vi "Evaluate Macro Command.vi"(8 "Error In":errorcluster, 10 "Cmd Index":i32, 11 "Macro Command String IN":string="LOOP.Start\t(loop.iterations,3.000);") -> (0 "Error Out":errorcluster, 1 "Warning?":bool, 2 "Macro Error Cluster":T1, 3 "Error in Command?":bool)   [LabVIEW 2012]
doc: "SciScan 1.2 160622"
uses:
  Macro Rule/subVIs/Error Checking/Macro Error Cluster.ctl
  INI/settingsIO/Settings IO_Commands.ctl
  FGV_MacroCore_Commands.ctl
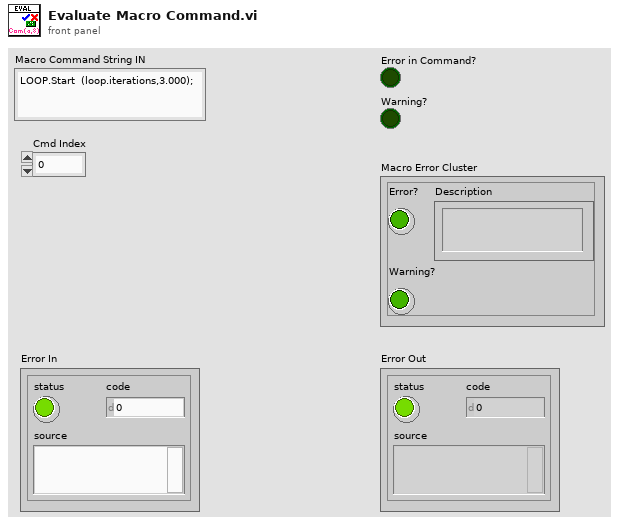
[diagram p1: front panel]
types:
  T1 = typedef "Macro Error Cluster.ctl" = cluster{"Error?":bool, "Description":string, "Warning?":bool}
  T2 = typedef "Settings IO_Commands.ctl" = enum16{"Write HW Settings", "Write Config Settings", "Read HW Settings", "Read Config Settings", "Write Line-Scan Settings", "Write Frame-Scan Settings", "Write Z-Stack Settings", "Read Line-Scan Settings", "Read Frame-Scan Settings", "Read Z-Stack Settings", "Read Fast-Z Settings", "Write Fast-Z Settings"}
  T3 = typedef "Macro_Action_List.ctl" = enum16{"Unknown Command", "2D.Frame.Scan", "2D.Line.Scan", "Load.Settings.File", "Move.To.Position", "Pause", "Z.Stack", "LOOP.Start", "LOOP.End", "Record", "Fast.Z", "Generic", "Slow.Z", "Tiling", "Preset.End"}
  T4 = typedef "GFG Variable for IO.ctl" = cluster{"Variable Name":string, "Value (Variant)":variant, "data type":string}
  T5 = typedef "FGV_MacroCore_Commands.ctl" = enum16{"Initialize", "Get Array", "Load macro from file", "Insert Item", "Insert at End", "Edit Parameter String", "Delete instruction", "Move Items", "Save", "SaveAs", "UpdateInfoTable", "Edit Settings File", "New Macro", "Read Temp File", "Delete Multiple"}
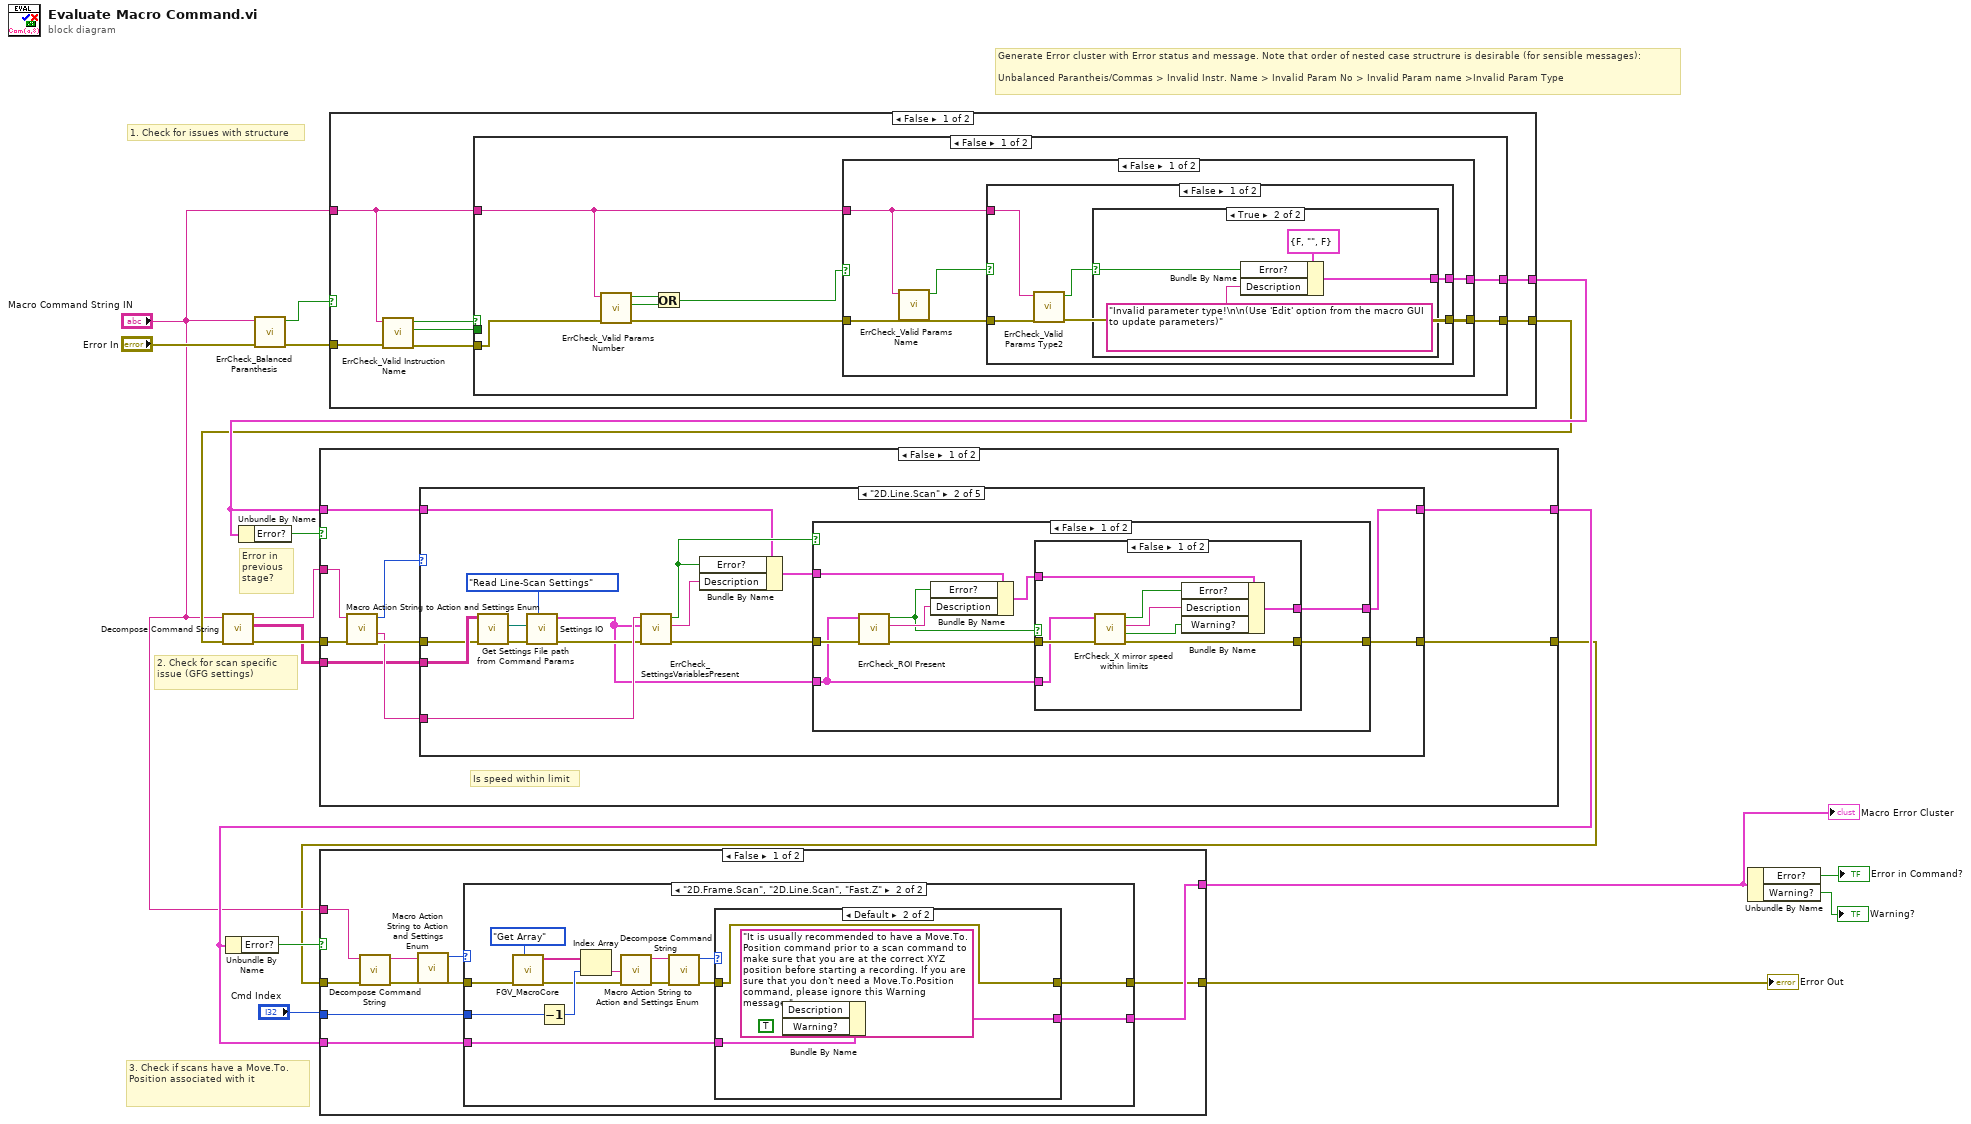
[diagram p0: block diagram]
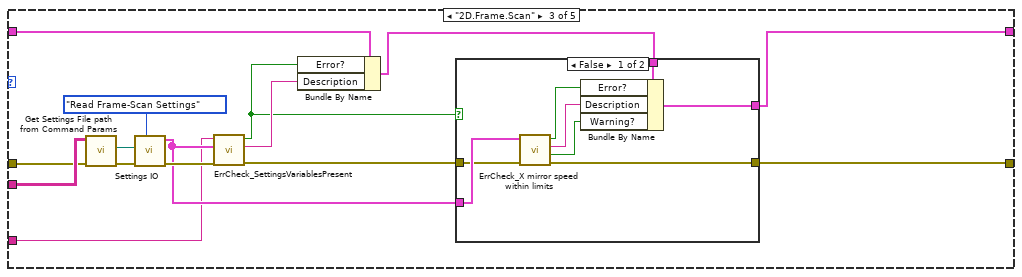
[diagram p8: hidden frame]
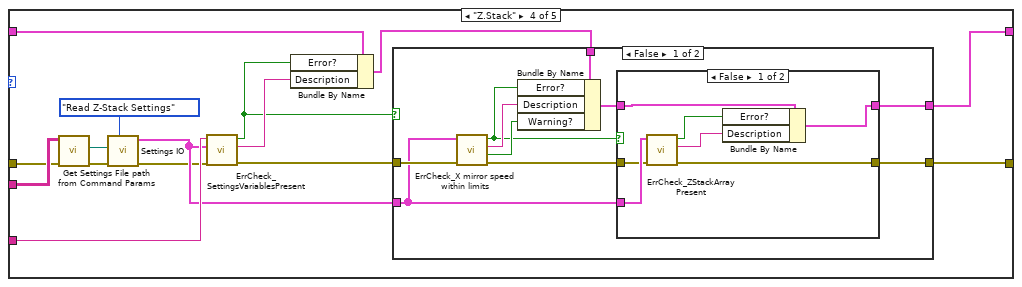
[diagram p10: hidden frame]
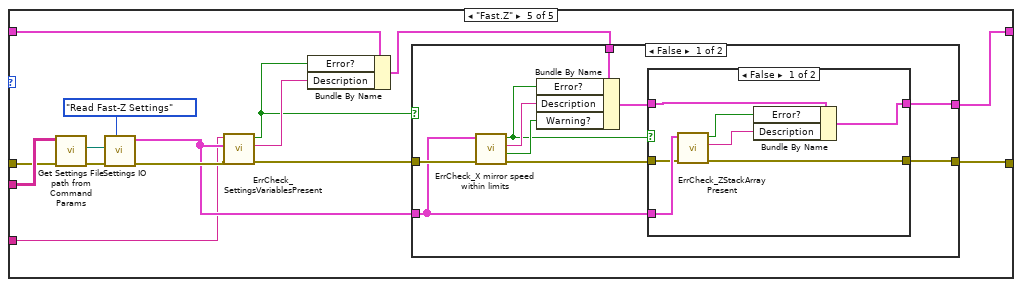
[diagram p13: hidden frame]
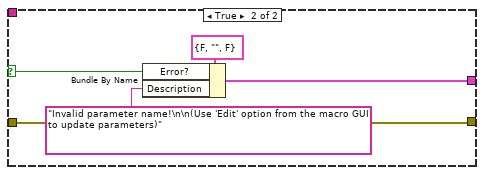
[diagram p18: hidden frame]
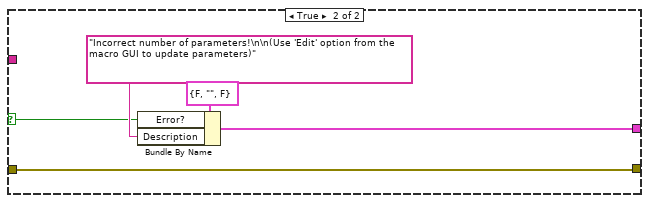
[diagram p19: hidden frame]
diagram:
  # "3. Check if scans have a Move.To.Position associated with it"
  # "2. Check for scan specific issue (GFG settings)"
  # "Error in previous stage?"
  # "1. Check for issues with structure"
  # "Generate Error cluster with Error status and message. Note that order of nested case structrure is desirable (for sensible messages):\n\nUnbalanced Parantheis/Commas > Invalid Instr. Name > Invalid Param No > Invalid Param name >Invalid Param Type"
  n1 = call "ErrCheck_Balanced Paranthesis.vi"("Error In"="Error In", "Macro Command String IN"="Macro Command String IN") -> ("Error Out"=w17:errorcluster, "Unbalanced Paranthesis or Commas?"=w16:bool)  [unwired: 8 in]
  n2 = case shown="False" w16 {
    selector: w16 -> [_ w68]
    tunnel: "Macro Command String IN" -> [w25 _]
    tunnel: [w24 w66] -> w11
    tunnel: w17 -> [w23 w66]
    tunnel: [w21 w67] -> w13
    frame False {
      n3 = call "ErrCheck_Valid Instruction Name.vi"("Error In"=w23, "Macro Command String IN"=w25) -> ("Error Out"=w22:errorcluster, "Generic Instruction?"=w20:bool, "Invalid Instruction name?"=w19:bool)  [unwired: 7 in]
      n4 = case shown="False" w19 {
        selector: w19 -> [_ w60]
        tunnel: w25 -> [w33 _]
        tunnel: [w31 w58] -> w24
        tunnel: w22 -> [w30 w58]
        tunnel: [w26 w61] -> w21
        tunnel: w20 -> [_ w59]
        frame False {
          n5 = call "ErrCheck_Valid Params Number.vi"("Error In"=w30, "Macro Command String IN"=w33) -> ("Error Out"=w27:errorcluster, "Less params than expected?"=w28:bool, "More params than expected?"=w29:bool)  [unwired: 7 in]
          n6 = Or(x=w29, y=w28) -> (x .or. y?=w32:bool)
          n7 = case shown="False" w32 {
            selector: w32 -> [_ w55]
            tunnel: w33 -> [w34 _]
            tunnel: [w38 w53] -> w31
            tunnel: w27 -> [w37 w53]
            tunnel: [w35 w54] -> w26
            frame False {
              n8 = call "ErrCheck_Valid Params Name.vi"("Macro Command String IN"=w34) -> ("Invalid Params name?"=w36:bool)  [unwired: 9 in, 1 out]
              n9 = case shown="False" w36 {
                selector: w36 -> [_ w50]
                tunnel: w34 -> [w43 _]
                tunnel: [w42 w48] -> w38
                tunnel: w37 -> [w41 w48]
                tunnel: [w39 w49] -> w35
                frame False {
                  n10 = call "ErrCheck_Valid Params Type2.vi"("Error In"=w41, "Macro Command String IN"=w43) -> ("Error Out"=w42:errorcluster, "Invalid params type?"=w40:bool)  [unwired: 8 in]
                  n11 = case shown="True" w40 {
                    selector: w40 -> [_ w45]
                    tunnel: [_ w44] -> w39
                    frame False {
                    }
                    frame True {
                      n12 = Bundle By Name(cluster=T1 {"Error?"=FALSE, "Description"="", "Warning?"=FALSE} ("Macro Error Cluster"), "Error?"=w45, "Description"="Invalid parameter type!\n\n(Use 'Edit' option from the macro GUI to update parameters)") -> (w44:T1)
                    }
                  }
                }
                frame True {
                  n13 = Bundle By Name(cluster=T1 {"Error?"=FALSE, "Description"="", "Warning?"=FALSE} ("Macro Error Cluster"), "Error?"=w50, "Description"="Invalid parameter name!\n\n(Use 'Edit' option from the macro GUI to update parameters)") -> (w49:T1)
                }
              }
            }
            frame True {
              n14 = Bundle By Name(cluster=T1 {"Error?"=FALSE, "Description"="", "Warning?"=FALSE} ("Macro Error Cluster"), "Error?"=w55, "Description"="Incorrect number of parameters!\n\n(Use 'Edit' option from the macro GUI to update parameters)") -> (w54:T1)
            }
          }
        }
        frame True {
          n15 = case shown="True" w59 {
            tunnel: [w65 _] -> w61
            tunnel: w60 -> [w62 _]
            frame False {
              n16 = Bundle By Name(cluster=T1 {"Error?"=FALSE, "Description"="", "Warning?"=FALSE} ("Macro Error Cluster"), "Error?"=w62, "Description"="Invalid instruction name!\n\nDelete the instruction (drag and drop it into available actions), and add the instruction you want again") -> (w65:T1)
            }
            frame True {
            }
          }
        }
      }
    }
    frame True {
      n17 = Bundle By Name(cluster=T1 {"Error?"=FALSE, "Description"="", "Warning?"=FALSE} ("Macro Error Cluster"), "Error?"=w68, "Description"="Unbalanced parantheis or 'parameter-value' pairs!\n\n(Use 'Edit' option from the macro GUI to update parameters)") -> (w67:T1)
    }
  }
  n18 = call "Decompose Command String.vi"("Error In"=w11, "Command IN"="Macro Command String IN") -> ("Error Out"=w10:errorcluster, "Parameter Table"=w9:string[][], "Action"=w12:string)  [unwired: 6 in, 1 out]
  n19 = Unbundle By Name(w13) -> ("Error?"=w14:bool)
  n20 = case shown="False" w14 {
    tunnel: w10 -> [w77 w215]
    tunnel: w12 -> [w76 _]
    tunnel: w13 -> [w78 w216]
    tunnel: [w79 w216] -> w6
    tunnel: w9 -> [w72 _]
    tunnel: [w71 w215] -> w3
    frame False {
      # "Is speed within limit"
      n21 = call "Macro Action String to Action and Settings Enum.vi"("error in (no error)"=w77, "Action String IN"=w76) -> ("error out"=w74:errorcluster, "Settings File Type OUT (String)"=w73:string, "Action Enum OUT"=w75:T3)  [unwired: 6 in, 1 out]
      n22 = case shown="\"2D.Line.Scan\"" w75 {
        tunnel: [w81 w83 w127 w145 w180] -> w79
        tunnel: w78 -> [w81 w86 w120 w146 w182]
        tunnel: w74 -> [w80 w92 w128 w153 w189]
        tunnel: w73 -> [_ w91 w122 w148 w181]
        tunnel: w72 -> [_ w95 w131 w156 w192]
        tunnel: [w80 w82 w126 w144 w179] -> w71
        frame "Unknown Command", Default {
        }
        frame "2D.Line.Scan" {
          n23 = call "Get Settings File path from Command Params.vi"("error in (no error)"=w92, "Params Array IN"=w95) -> ("error out"=w93:errorcluster, "Settings Path OUT"=w94:path)  [unwired: 8 in]
          n24 = call "Settings IO.vi"("SettingsFileIO_Commands"=Settings_IO_Commands."Read Line-Scan Settings", "Error In"=w93, "File Path (for scan specific settings)"=w94) -> ("Error Out"=w89:errorcluster, "Settings Array OUT"=w87:T4[])  [unwired: 6 in, 1 out]
          n25 = call "ErrCheck_SettingsVariablesPresent.vi"("error in (no error)"=w89, "Settings Array IN"=w87, "Settings type string"=w91) -> ("error out"=w84:errorcluster, "Error String"=w90:string, "Error?"=w88:bool)  [unwired: 6 in]
          n26 = Bundle By Name(cluster=w86, "Error?"=w88, "Description"=w90) -> (w85:T1)
          n27 = case shown="False" w88 {
            tunnel: w87 -> [w99 _]
            tunnel: w85 -> [w104 w117]
            tunnel: w84 -> [w101 w116]
            tunnel: [w98 w117] -> w83
            tunnel: [w97 w116] -> w82
            frame False {
              n28 = call "ErrCheck_ROI Present.vi"("Error In"=w101, "Settings ArrayIN"=w99) -> ("Error Out"=w100:errorcluster, "Error/Warning Message"=w105:string, "ROI Descriptor Missing?"=w103:bool)  [unwired: 7 in]
              n29 = Bundle By Name(cluster=w104, "Error?"=w103, "Description"=w105) -> (w102:T1)
              n30 = case shown="False" w103 {
                tunnel: w102 -> [w110 w115]
                tunnel: w100 -> [w109 w114]
                tunnel: w99 -> [w108 _]
                tunnel: [w107 w115] -> w98
                tunnel: [w106 w114] -> w97
                frame False {
                  n31 = call "ErrCheck_X mirror speed within limits.vi"("Error In"=w109, "Settings ArrayIN"=w108) -> ("Error Out"=w106:errorcluster, "Not Enough Variables (Warning)?"=w112:bool, "Error/Warning Message"=w113:string, "Speed  out of Limits?"=w111:bool)  [unwired: 6 in]
                  n32 = Bundle By Name(cluster=w110, "Error?"=w111, "Description"=w113, "Warning?"=w112) -> (w107:T1)
                }
                frame True {
                }
              }
            }
            frame True {
            }
          }
        }
        frame "2D.Frame.Scan" {
          n33 = call "Get Settings File path from Command Params.vi"("error in (no error)"=w128, "Params Array IN"=w131) -> ("error out"=w129:errorcluster, "Settings Path OUT"=w130:path)  [unwired: 8 in]
          n34 = call "Settings IO.vi"("SettingsFileIO_Commands"=Settings_IO_Commands."Read Frame-Scan Settings", "Error In"=w129, "File Path (for scan specific settings)"=w130) -> ("Error Out"=w124:errorcluster, "Settings Array OUT"=w123:T4[])  [unwired: 6 in, 1 out]
          n35 = call "ErrCheck_SettingsVariablesPresent.vi"("error in (no error)"=w124, "Settings Array IN"=w123, "Settings type string"=w122) -> ("error out"=w121:errorcluster, "Error String"=w125:string, "Error?"=w118:bool)  [unwired: 6 in]
          n36 = Bundle By Name(cluster=w120, "Error?"=w118, "Description"=w125) -> (w119:T1)
          n37 = case shown="False" w118 {
            tunnel: w121 -> [w136 w141]
            tunnel: w123 -> [w137 _]
            tunnel: w119 -> [w134 w142]
            tunnel: [w133 w142] -> w127
            tunnel: [w135 w141] -> w126
            frame False {
              n38 = call "ErrCheck_X mirror speed within limits.vi"("Error In"=w136, "Settings ArrayIN"=w137) -> ("Error Out"=w135:errorcluster, "Not Enough Variables (Warning)?"=w139:bool, "Error/Warning Message"=w138:string, "Speed  out of Limits?"=w140:bool)  [unwired: 6 in]
              n39 = Bundle By Name(cluster=w134, "Error?"=w140, "Description"=w138, "Warning?"=w139) -> (w133:T1)
            }
            frame True {
            }
          }
        }
        frame "Z.Stack" {
          n40 = call "Get Settings File path from Command Params.vi"("error in (no error)"=w153, "Params Array IN"=w156) -> ("error out"=w154:errorcluster, "Settings Path OUT"=w155:path)  [unwired: 8 in]
          n41 = call "Settings IO.vi"("SettingsFileIO_Commands"=Settings_IO_Commands."Read Z-Stack Settings", "Error In"=w154, "File Path (for scan specific settings)"=w155) -> ("Error Out"=w143:errorcluster, "Settings Array OUT"=w147:T4[])  [unwired: 6 in, 1 out]
          n42 = call "ErrCheck_SettingsVariablesPresent.vi"("error in (no error)"=w143, "Settings Array IN"=w147, "Settings type string"=w148) -> ("error out"=w151:errorcluster, "Error String"=w152:string, "Error?"=w149:bool)  [unwired: 6 in]
          n43 = Bundle By Name(cluster=w146, "Error?"=w149, "Description"=w152) -> (w150:T1)
          n44 = case shown="False" w149 {
            tunnel: w151 -> [w165 w177]
            tunnel: w147 -> [w160 _]
            tunnel: w150 -> [w164 w178]
            tunnel: [w161 w178] -> w145
            tunnel: [w158 w177] -> w144
            frame False {
              n45 = call "ErrCheck_X mirror speed within limits.vi"("Error In"=w165, "Settings ArrayIN"=w160) -> ("Error Out"=w159:errorcluster, "Not Enough Variables (Warning)?"=w167:bool, "Error/Warning Message"=w166:string, "Speed  out of Limits?"=w163:bool)  [unwired: 6 in]
              n46 = Bundle By Name(cluster=w164, "Error?"=w163, "Description"=w166, "Warning?"=w167) -> (w162:T1)
              n47 = case shown="False" w163 {
                tunnel: w162 -> [w172 w176]
                tunnel: [w168 w176] -> w161
                tunnel: w160 -> [w174 _]
                tunnel: w159 -> [w173 w175]
                tunnel: [w169 w175] -> w158
                frame False {
                  n48 = call "ErrCheck_ZStackArray Present.vi"("Error In"=w173, "Settings ArrayIN"=w174) -> ("Error Out"=w169:errorcluster, "Error/Warning Message"=w170:string, "Z-Stack data missing?"=w171:bool)  [unwired: 7 in]
                  n49 = Bundle By Name(cluster=w172, "Error?"=w171, "Description"=w170) -> (w168:T1)
                }
                frame True {
                }
              }
            }
            frame True {
            }
          }
        }
        frame "Fast.Z" {
          n50 = call "Get Settings File path from Command Params.vi"("error in (no error)"=w189, "Params Array IN"=w192) -> ("error out"=w190:errorcluster, "Settings Path OUT"=w191:path)  [unwired: 8 in]
          n51 = call "Settings IO.vi"("SettingsFileIO_Commands"=Settings_IO_Commands."Read Fast-Z Settings", "Error In"=w190, "File Path (for scan specific settings)"=w191) -> ("Error Out"=w184:errorcluster, "Settings Array OUT"=w183:T4[])  [unwired: 6 in, 1 out]
          n52 = call "ErrCheck_SettingsVariablesPresent.vi"("error in (no error)"=w184, "Settings Array IN"=w183, "Settings type string"=w181) -> ("error out"=w187:errorcluster, "Error String"=w188:string, "Error?"=w185:bool)  [unwired: 6 in]
          n53 = Bundle By Name(cluster=w182, "Error?"=w185, "Description"=w188) -> (w186:T1)
          n54 = case shown="False" w185 {
            tunnel: w187 -> [w201 w213]
            tunnel: w183 -> [w198 _]
            tunnel: w186 -> [w200 w214]
            tunnel: [w196 w214] -> w180
            tunnel: [w195 w213] -> w179
            frame False {
              n55 = call "ErrCheck_X mirror speed within limits.vi"("Error In"=w201, "Settings ArrayIN"=w198) -> ("Error Out"=w199:errorcluster, "Not Enough Variables (Warning)?"=w203:bool, "Error/Warning Message"=w202:string, "Speed  out of Limits?"=w194:bool)  [unwired: 6 in]
              n56 = Bundle By Name(cluster=w200, "Error?"=w194, "Description"=w202, "Warning?"=w203) -> (w197:T1)
              n57 = case shown="False" w194 {
                tunnel: w197 -> [w208 w212]
                tunnel: [w204 w212] -> w196
                tunnel: w198 -> [w210 _]
                tunnel: w199 -> [w209 w211]
                tunnel: [w205 w211] -> w195
                frame False {
                  n58 = call "ErrCheck_ZStackArray Present.vi"("Error In"=w209, "Settings ArrayIN"=w210) -> ("Error Out"=w205:errorcluster, "Error/Warning Message"=w206:string, "Z-Stack data missing?"=w207:bool)  [unwired: 7 in]
                  n59 = Bundle By Name(cluster=w208, "Error?"=w207, "Description"=w206) -> (w204:T1)
                }
                frame True {
                }
              }
            }
            frame True {
            }
          }
        }
      }
    }
    frame True {
    }
  }
  n60 = Unbundle By Name(w6) -> ("Error?"=w7:bool)
  n61 = case shown="False" w7 {
    tunnel: [w218 w251] -> w2
    tunnel: w6 -> [w219 w251]
    tunnel: "Cmd Index" -> [w226 _]
    tunnel: "Macro Command String IN" -> [w225 _]
    tunnel: w3 -> [w221 w250]
    tunnel: [w217 w250] -> w1
    frame False {
      n62 = call "Decompose Command String.vi"("Error In"=w221, "Command IN"=w225) -> ("Error Out"=w222:errorcluster, "Action"=w224:string)  [unwired: 6 in, 2 out]
      n63 = call "Macro Action String to Action and Settings Enum.vi"("error in (no error)"=w222, "Action String IN"=w224) -> ("error out"=w220:errorcluster, "Action Enum OUT"=w223:T3)  [unwired: 6 in, 2 out]
      n64 = case shown="\"2D.Frame.Scan\", \"2D.Line.Scan\", \"Fast.Z\"" w223 {
        tunnel: w226 -> [_ w240]
        tunnel: w220 -> [w227 w238]
        tunnel: w219 -> [w228 w234]
        tunnel: [w228 w233] -> w218
        tunnel: [w227 w230] -> w217
        frame "Unknown Command", Default {
        }
        frame "2D.Frame.Scan", "2D.Line.Scan", "Fast.Z" {
          n65 = call "FGV_MacroCore.vi"("MacroFGV_Commands"=FGV_MacroCore_Commands."Get Array", "Error In"=w238) -> ("Error Out"=w236:errorcluster, "Macro String Array"=w241:string[])  [unwired: 5 in, 3 out]
          n66 = Decrement(x=w240) -> (x-1=w239:i32)
          n67 = Index Array(array=w241, index=w239) -> (element=w237:string)
          n68 = call "Decompose Command String.vi"("Error In"=w236, "Command IN"=w237) -> ("Error Out"=w231:errorcluster, "Action"=w232:string)  [unwired: 6 in, 2 out]
          n69 = call "Macro Action String to Action and Settings Enum.vi"("error in (no error)"=w231, "Action String IN"=w232) -> ("error out"=w229:errorcluster, "Action Enum OUT"=w235:T3)  [unwired: 6 in, 2 out]
          n70 = case shown="Default" w235 {
            tunnel: w234 -> [w244 w249]
            tunnel: [w244 w246] -> w233
            tunnel: [w243 w245] -> w230
            tunnel: w229 -> [w243 w245]
            frame "Move.To.Position" {
            }
            frame Default {
              n71 = Bundle By Name(cluster=w249, "Description"="It is usually recommended to have a Move.To.Position command prior to a scan command to make sure that you are at the correct XYZ position before starting a recording. If you are sure that you don't need a Move.To.Position command, please ignore this Warning message.", "Warning?"=TRUE) -> (w246:T1)
            }
          }
        }
      }
    }
    frame True {
    }
  }
  "Error Out" <- w1
  "Macro Error Cluster" <- w2
  n72 = Unbundle By Name(w2) -> ("Error?"=→"Error in Command?":bool, "Warning?"=→"Warning?":bool)
